vi "Update Plugin Tree Save State.vi"(8 "error in (no error)":errorcluster, 11 "TreeControl in":refnum<vi>) -> (0 "error out":errorcluster, 3 "TreeControl out":refnum<vi>)   [LabVIEW 2018]
uses:
  Queue/Queue.lvlib
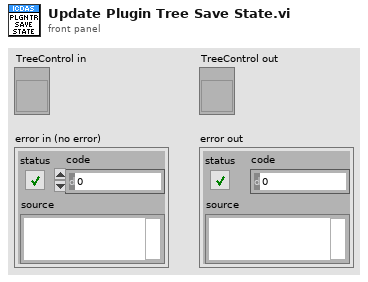
[diagram p1: front panel]
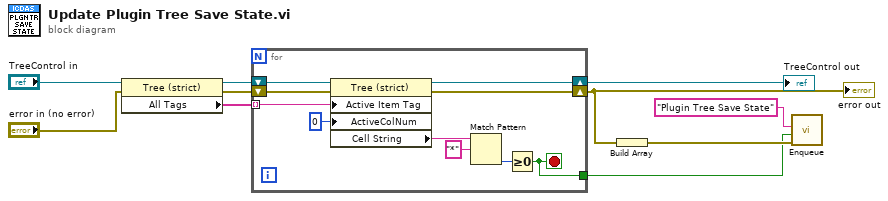
[diagram p0: block diagram]
diagram:
  n1 = property class="Tree (strict)"(reference="TreeControl in", error in="error in (no error)") -> (reference out=w7:refnum<vi>, error out=w8:errorcluster, "All Tags"=w6:string[])
  n2 = for {
    shift-right: [w19] -> w4
    shift-left: w7 -> [w20]
    shift-right: [w12] -> w3
    shift-left: w8 -> [w18]
    tunnel: w6 -> [w17] mode=indexing
    tunnel: [w11] -> w1
    stop <- w11 stop-if-true
    n3 = property class="Tree (strict)"(reference=w20, error in=w18, "Active Item Tag"=w17, "ActiveColNum"=0 ("Active Cell:Active Column Number")) -> (reference out=w19:refnum<vi>, error out=w12:errorcluster, "Cell String"=w15:string)
    n4 = Match Pattern(string=w15, regular expression="*") -> (offset past match=w13:i32)  [unwired: 1 in, 3 out]
    n5 = Greater Or Equal To 0?(x=w13) -> (x >= 0?=w11:bool)
  }
  "error out" <- w3
  "TreeControl out" <- w4
  n6 = Build Array(w3) -> (w5:errorcluster[])
  n7 = call "Enqueue.vi"("ErrorArray"=w5, "Message Data"=w1, "Message"="Plugin Tree Save State") -> ()  [unwired: 8 in, 1 out]
